vi "_FPGA Read ADC.vi"(6 "error in":errorcluster, 8 "ADC Channel (64)":u8=64) -> (0 "error out":errorcluster, 1 "Running":bool, 2 "User Value":sgl, 3 "ADC Values":i32[](array[numeric]), 4 "In Range?":bool, 5 "Raw Reading":sgl)   [LabVIEW 2012]
uses:
  Type/_FPGA Indicator.ctl
  _RT Global.vi
  <vilib>/Utility/error.llb/Error Cluster From Error Code.vi
  <vilib>/rvi/errors/niLvFpgaAdjustHostInterfaceError.vi
  <vilib>/rvi/interface/nirviReadWriteControl/nirviReadWriteControl.xnode
  FPGA Bitfiles/FPGA9606.lvbitx
  NiFpgaLv.dll
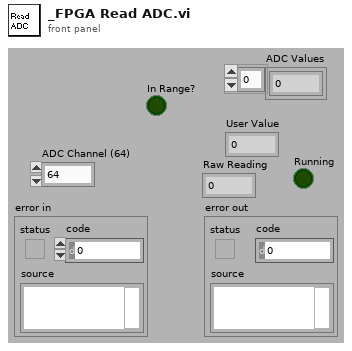
[diagram p1: front panel]
types:
  T1 = typedef "Semaphore RefNum" = refnum<k1>
  T2 = typedef "_FPGA Indicator.ctl" = enum16{"Done", "Ready", "Count Available", "SendSerial", "LED State"}
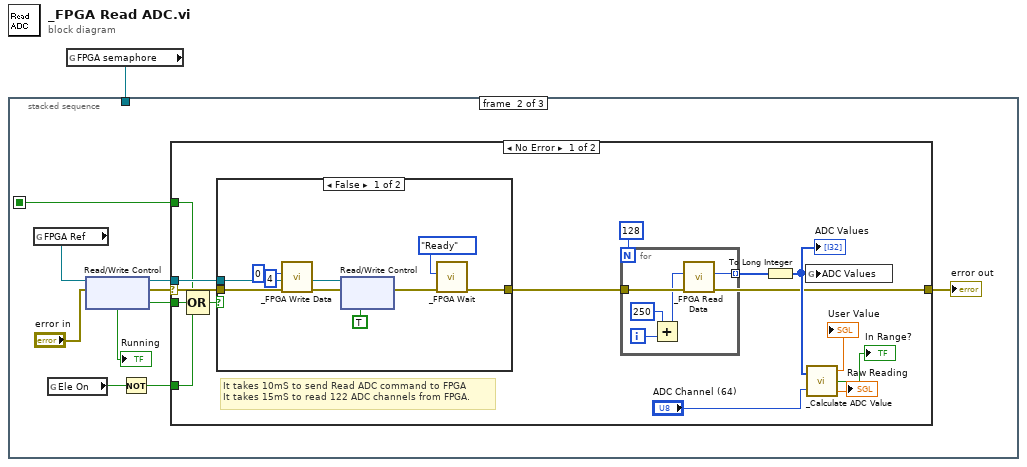
[diagram p0: block diagram]
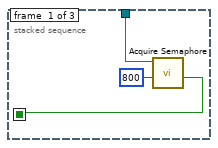
[diagram p2: hidden frame]
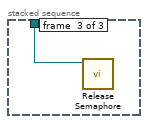
[diagram p5: hidden frame]
diagram:
  n1 = global read "_RT Global.vi" "FPGA semaphore"() -> (w1:T1)
  n2 = stacked-sequence {
    seq-local: [w2 _ _] -> [_ w6 _]
    tunnel: w1 -> [w4 _ w44]
    frame #0 {
      n3 = call <vilib>:"Acquire Semaphore.vi"("ms timeout (-1)"=800, "semaphore"=w4) -> ("timed out"=w2:bool)  [unwired: 1 in, 4 out]
    }
    frame #1 {
      n4 = global read "_RT Global.vi" "FPGA Ref"() -> (w5:refnum<k20>)
      n5 = global read "_RT Global.vi" "Ele On"() -> (w8:bool)
      n6 = xnode "Read/Write Control"("FPGA VI Reference In"=w5, "error in"="error in") -> ("FPGA VI Reference Out"=w11:refnum<k20>, "error out"=w12:errorcluster, "Running"=w9:bool)
      "Running" <- w9
      n7 = Not(x=w8) -> (.not. x?=w7:bool)
      n8 = case shown="No Error" w12 {
        selector: w12 -> [w27 w43]
        tunnel: [w14 w43] -> w13
        tunnel: w11 -> [w26 _]
        tunnel: w9 -> [w20 _]
        tunnel: w7 -> [w17 _]
        tunnel: w6 -> [w15 _]
        frame No Error {
          # "It takes 10mS to send Read ADC command to FPGA\nIt takes 15mS to read 122 ADC channels from FPGA."
          n9 = Compound Arithmetic op=OR(w15, w20, w17) -> (w18:bool)
          n10 = case shown="False" w18 {
            tunnel: [w38 w42] -> w14
            tunnel: w27 -> [w40 w42]
            tunnel: w26 -> [w39 _]
            frame False {
              n11 = call "_FPGA Write Data.vi"("error in"=w40, "Data"=u32 4 ("Address"), "Address"=u16 0) -> ("error out"=w37:errorcluster)  [unwired: 3 in, 2 out]
              n12 = xnode "Read/Write Control"("FPGA VI Reference In"=w39, "error in"=w37, "Start"=TRUE) -> ("error out"=w41:errorcluster)  [unwired: 1 out]
              n13 = call "_FPGA Wait.vi"("error in"=w41, "Indicator"=_FPGA_Indicator."Ready") -> ("error out"=w38:errorcluster)  [unwired: 3 in, 2 out]
            }
            frame True {
            }
          }
          n14 = for {
            N: 128 -> [_]
            tunnel: [w29] -> w22 mode=indexing
            tunnel: w14 -> [w28]
            i -> [w30]
            n15 = Add(x=250, y=w30) -> (x+y=w31:i32)
            n16 = call "_FPGA Read Data.vi"("error in"=w28, "Address"=w31) -> ("Data"=w29:u32)  [unwired: 3 in, 2 out]
          }
          n17 = To Long Integer(number=w22) -> (32bit integer=w21:i32[])
          "ADC Values" <- w21
          n18 = global write "_RT Global.vi" "ADC Values"(w21) -> ()
          n19 = call "_Calculate ADC Value.vi"("ADC Values"=w21, "ADC Channel (64)"="ADC Channel (64)") -> ("User Value"=→"User Value":sgl, "In Range?"=→"In Range?":bool, "Raw Reading"=→"Raw Reading":sgl)
        }
        frame Error {
        }
      }
      "error out" <- w13
    }
    frame #2 {
      n20 = call <vilib>:"Release Semaphore.vi"("semaphore"=w44) -> ()  [unwired: 1 in, 6 out]
    }
  }
